vi "Main.vi"() -> ()   [LabVIEW 2024]
doc: "This template is for the Queued Message Handler design pattern.\n\nThe Event Handling Loop generates messages based on user interface actions.\n\nThe Message Handling Loop processes messages generated by the Event Handling Loop, or by other messages. The messages are string values, so new messages can be added easily to the Message Cases case structure in the Message Handling Loop. Each message cluster can also provide an optional value for Message Data, which is a variant that can be converted to whatever message-specific data is required."
uses:
  controls/UI Data.ctl
  support/Message Queue/Enqueue Message (Single).vi
  <vilib>/Utility/error.llb/Error Cluster From Error Code.vi
  <vilib>/ErrorRing/Error Ring.xnode
  support/Message Queue/Message Queue.lvlib
  support/User Event - Stop/User Event - Stop.lvlib
  01 Queues/User Events.lvlib
panel:
  out "Waveform Chart":dbl(graph)
  in  "Knob":dbl(knob) scale=0.0..10.0
  out "Letrero":string
  in  "Hacer otra Cosa":bool
  in  "Hacer Algo":bool
  in  "Sali":bool
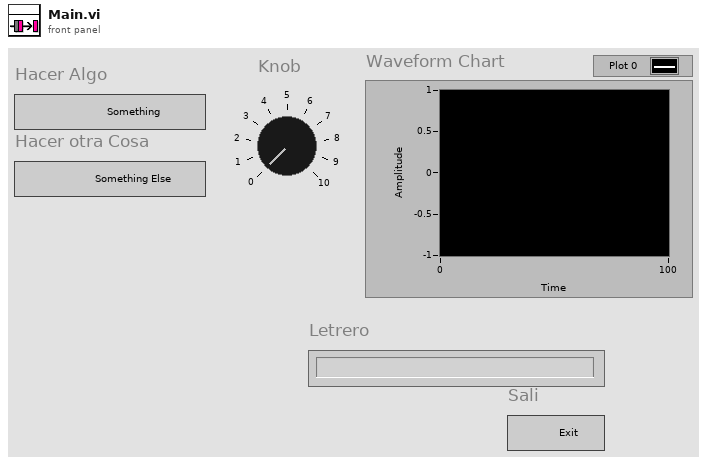
[diagram p1: front panel]
types:
  T1 = typedef "UI Data.ctl" = cluster{"Boolean <Replace Me>":bool, "String <Replace Me>":string, "Numeric <Replace Me>":dbl, "Do Something Ref":refnum<vi>, "Do Something Else Ref":refnum<vi>, "Data Display Ref":refnum<vi>, "Exit Button Ref":refnum<vi>}
  T2 = typedef "Message Queue.lvlib/All Message Queues.ctl" = cluster{"UI":refnum<queue>}
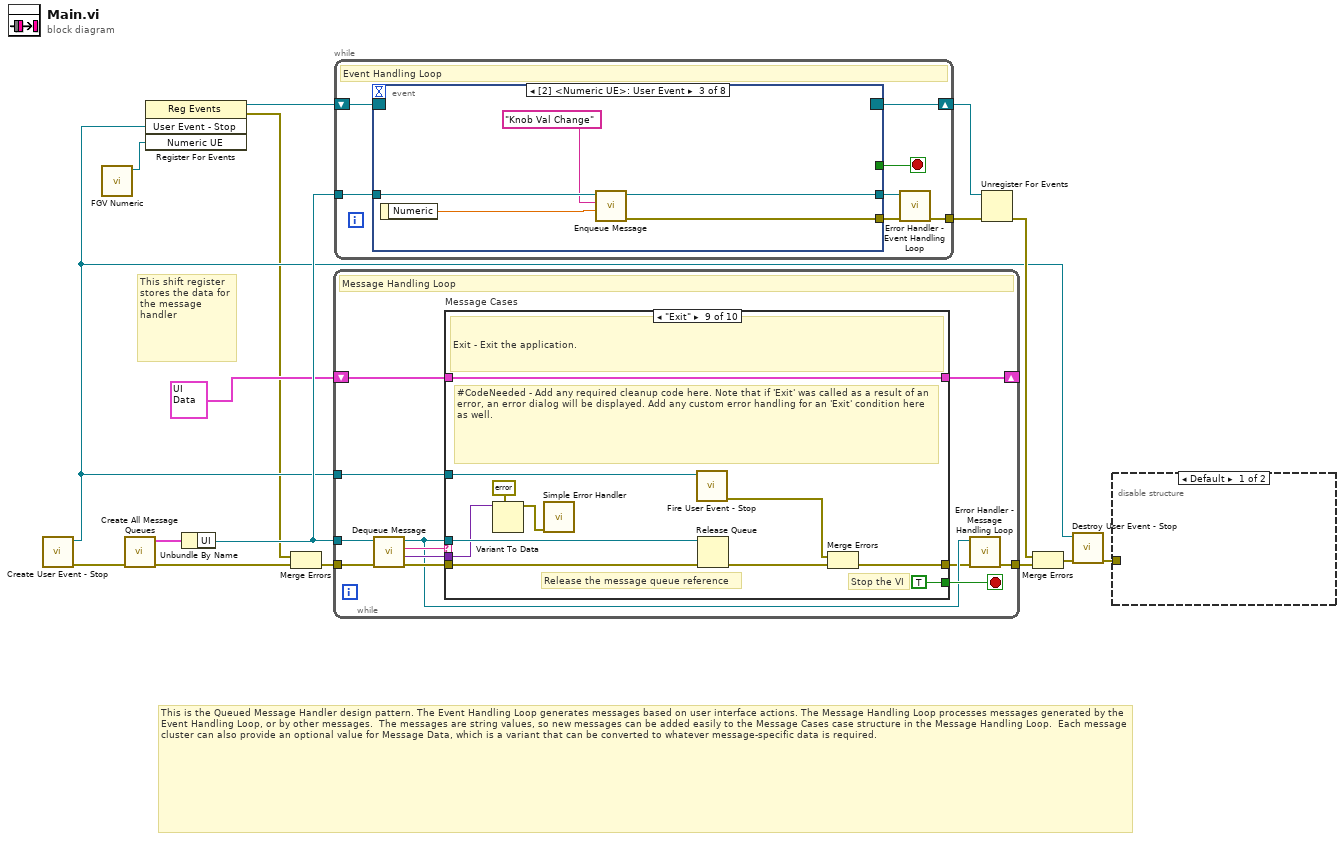
[diagram p0: block diagram]
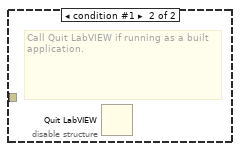
[diagram p2: hidden frame]
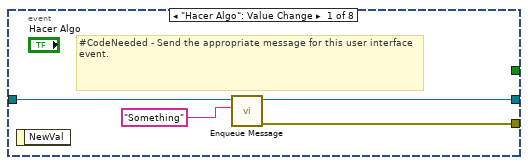
[diagram p3: hidden frame]
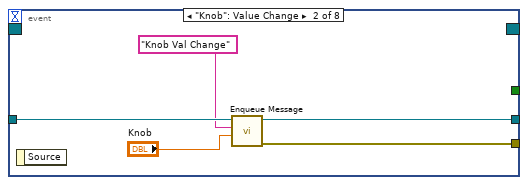
[diagram p4: hidden frame]
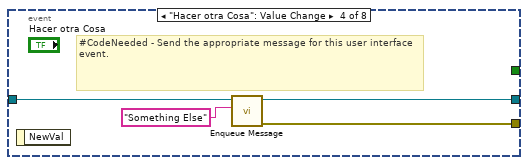
[diagram p5: hidden frame]
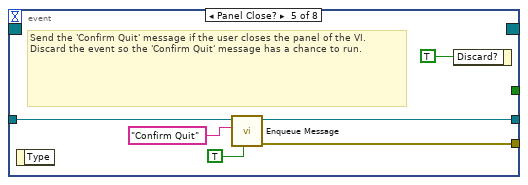
[diagram p6: hidden frame]
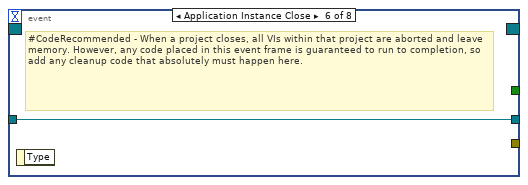
[diagram p7: hidden frame]
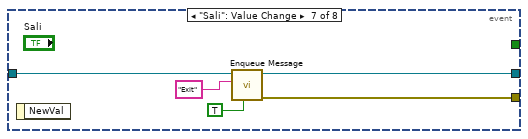
[diagram p8: hidden frame]
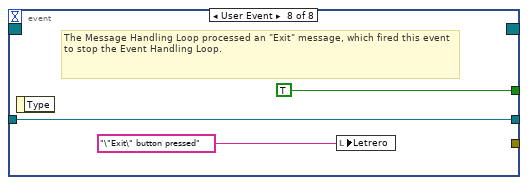
[diagram p9: hidden frame]
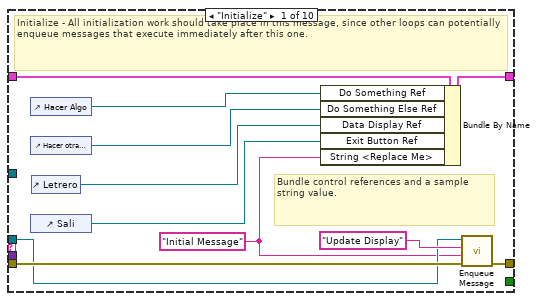
[diagram p10: hidden frame]
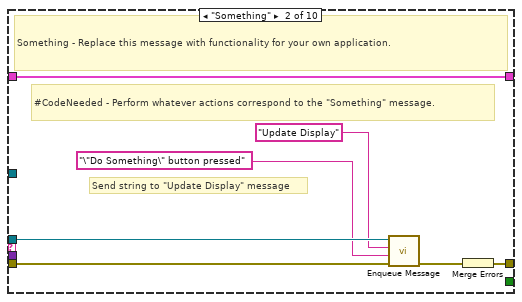
[diagram p11: hidden frame]
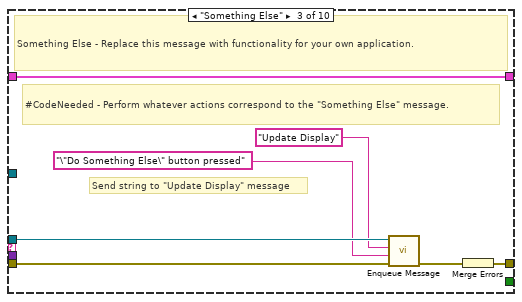
[diagram p12: hidden frame]
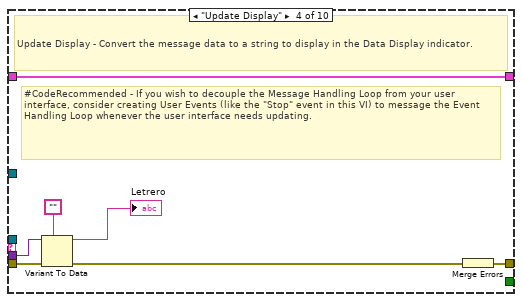
[diagram p13: hidden frame]
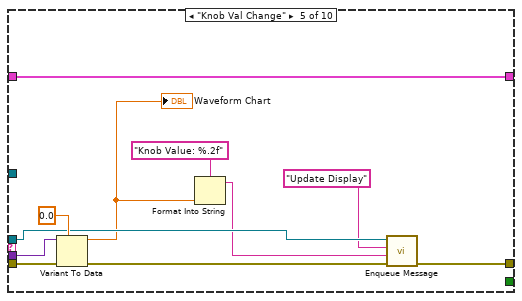
[diagram p14: hidden frame]
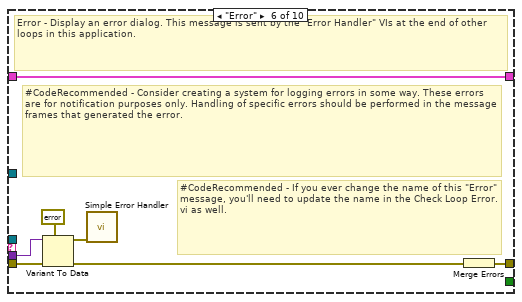
[diagram p15: hidden frame]
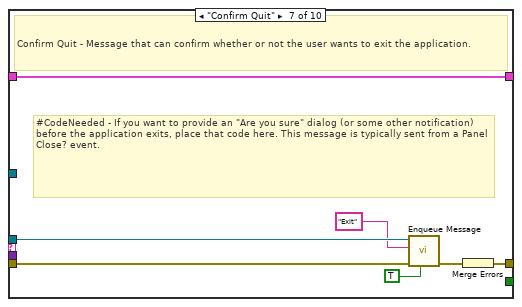
[diagram p16: hidden frame]
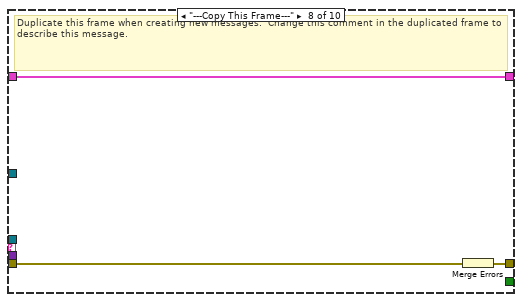
[diagram p17: hidden frame]
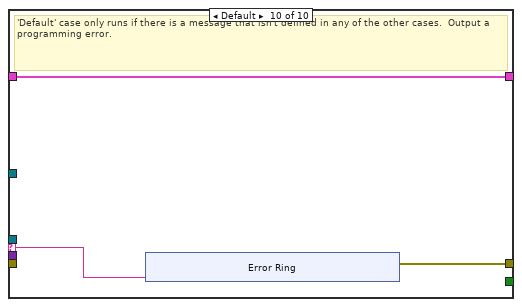
[diagram p18: hidden frame]
diagram:
  # "This is the Queued Message Handler design pattern. The Event Handling Loop generates messages based on user interface actions. The Message Handling Loop processes messages generated by the Event Handling Loop, or by other messages.  The messages are string values, so new messages can be added easily to the Message Cases case structure in the Message Handling Loop.  Each message cluster can also provide an optional value for Message Data, which is a variant that can be converted to whatever message-specific data is required."
  # "This shift register stores the data for the message handler"
  n1 = call "Create User Event - Stop.vi"() -> ("error out"=w12:errorcluster, "User Event - Stop"=w4:refnum<user-event>)  [unwired: 10 in]
  n2 = call "FGV Numeric.vi"() -> ("Numeric UE"=w1:refnum<user-event>)  [unwired: 11 in]
  n3 = call "Create All Message Queues.vi"("error in (no error)"=w12) -> ("error out"=w16:errorcluster, "Message Queues out"=w15:T2)  [unwired: 9 in]
  n4 = register-events(w4, w1) -> (reference out=w5:refnum<event-registration>, error out=w2:errorcluster)  [unwired: 2 in]
  n5 = Unbundle By Name(w15) -> ("UI"=w13:refnum<queue>)
  n6 = Merge Errors(w2, w16) -> (w3:errorcluster)
  n7 = while {
    tunnel: w13 -> [w20]
    shift-right: [w27] -> _
    shift-left: T1 {"Boolean <Replace Me>"=FALSE, "String <Replace Me>"="", "Numeric <Replace Me>"=0.0, "Do Something Ref"=refnum, "Do Something Else Ref"=refnum, "Data Display Ref"=refnum, "Exit Button Ref"=refnum} ("Data Cluster") -> [w28]
    tunnel: w4 -> [w25]
    tunnel: w3 -> [w24]
    tunnel: [w18] -> w14
    stop <- w26 stop-if-true
    # "Message Handling Loop"
    n8 = call "Dequeue Message.vi"("error in (no error)"=w24, "Message Queue"=w20) -> ("error out"=w23:errorcluster, "Message Data"=w21:variant, "Message"=w22:string, "dup Message Queue"=w19:refnum<queue>)  [unwired: 6 in]
    n9 = case "Message Cases" shown="\"Exit\"" w22 {
      selector: w22 -> [_ _ _ _ _ _ _ _ _ w100]
      tunnel: w19 -> [w30 w42 w49 _ w65 _ w81 _ w99 _]
      tunnel: w23 -> [w38 w44 w51 w58 w71 w78 w85 w88 w92 _]
      tunnel: [w39 w45 w52 w59 w66 w72 w83 w86 w95 w101] -> w17
      tunnel: w28 -> [w37 w46 w53 w60 w70 w77 w84 w87 w98 w102]
      tunnel: [w36 w46 w53 w60 w70 w77 w84 w87 w98 w102] -> w27
      tunnel: [_ _ _ _ _ _ _ _ TRUE _] -> w26
      tunnel: w21 -> [_ _ _ w57 w68 w76 _ _ w89 _]
      tunnel: w25 -> [_ _ _ _ _ _ _ _ w94 _]
      frame "Initialize" {
        w29 = "Initial Message" ("Initial Message")
        # "Bundle control references and a sample string value."
        # "Initialize - All initialization work should take place in this message, since other loops can potentially enqueue messages that execute immediately after this one."
        n10 = control-ref of="Hacer Algo"() -> (w35:refnum<vi>)
        n11 = control-ref of="Hacer otra Cosa"() -> (w34:refnum<vi>)
        n12 = control-ref of="Sali"() -> (w32:refnum<vi>)
        n13 = control-ref of="Letrero"() -> (w33:refnum<vi>)
        n14 = Bundle By Name(cluster=w37, "Do Something Ref"=w35, "Do Something Else Ref"=w34, "Data Display Ref"=w33, "Exit Button Ref"=w32, "String <Replace Me>"=w29) -> (w36:T1)
        n15 = call-poly "Enqueue Message.vi"("error in (no error)"=w38, "Message Data"=w29, "Message"="Update Display", "Message Queue"=w30) -> ("error out"=w39:errorcluster)  [unwired: 6 in, 1 out]
      }
      frame "Something" {
        # "Send string to \"Update Display\" message"
        # "#CodeNeeded - Perform whatever actions correspond to the \"Something\" message."
        # "Something - Replace this message with functionality for your own application."
        n16 = call-poly "Enqueue Message.vi"("error in (no error)"=w44, "Message Data"="\"Do Something\" button pressed" ("\"Do Something\" button pressed"), "Message"="Update Display", "Message Queue"=w42) -> ("error out"=w43:errorcluster)  [unwired: 6 in, 1 out]
        n17 = Merge Errors(w43) -> (w45:errorcluster)
      }
      frame "Something Else" {
        # "Send string to \"Update Display\" message"
        # "#CodeNeeded - Perform whatever actions correspond to the \"Something Else\" message."
        # "Something Else - Replace this message with functionality for your own application."
        n18 = call-poly "Enqueue Message.vi"("error in (no error)"=w51, "Message Data"="\"Do Something Else\" button pressed" ("\"Do Something Else\" button pressed"), "Message"="Update Display", "Message Queue"=w49) -> ("error out"=w50:errorcluster)  [unwired: 6 in, 1 out]
        n19 = Merge Errors(w50) -> (w52:errorcluster)
      }
      frame "Update Display" {
        # "#CodeRecommended - If you wish to decouple the Message Handling Loop from your user interface, consider creating User Events (like the \"Stop\" event in this VI) to message the Event Handling Loop whenever the user interface needs updating."
        # "Update Display - Convert the message data to a string to display in the Data Display indicator."
        n20 = Variant To Data(error in=w58, type="", Variant=w57) -> (data=→"Letrero":string, error out=w55:errorcluster)
        n21 = Merge Errors(w55) -> (w59:errorcluster)
      }
      frame "Knob Val Change" {
        n22 = Variant To Data(error in=w71, type=0.0, Variant=w68) -> (data=w62:dbl, error out=w69:errorcluster)
        "Waveform Chart" <- w62
        n23 = Format Into String(format string="Knob Value: %.2f", w62) -> (resulting string=w63:string)  [unwired: 2 in, 1 out]
        n24 = call-poly "Enqueue Message.vi"("error in (no error)"=w69, "Message Data"=w63, "Message"="Update Display", "Message Queue"=w65) -> ("error out"=w66:errorcluster)  [unwired: 6 in, 1 out]
      }
      frame "Error" {
        # "#CodeRecommended - If you ever change the name of this \"Error\" message, you'll need to update the name in the Check Loop Error.vi as well."
        # "#CodeRecommended - Consider creating a system for logging errors in some way. These errors are for notification purposes only. Handling of specific errors should be performed in the message frames that generated the error."
        # "Error - Display an error dialog. This message is sent by the \"Error Handler\" VIs at the end of other loops in this application."
        n25 = Variant To Data(error in=w78, type=errorcluster {"status"=FALSE, "code"=0, "source"=""} ("error constant"), Variant=w76) -> (data=w74:errorcluster, error out=w73:errorcluster)
        n26 = call <vilib>:"Simple Error Handler.vi"("error in (no error)"=w74) -> ()  [unwired: 4 in, 5 out]
        n27 = Merge Errors(w73) -> (w72:errorcluster)
      }
      frame "Confirm Quit" {
        # "#CodeNeeded - If you want to provide an \"Are you sure\" dialog (or some other notification) before the application exits, place that code here. This message is typically sent from a Panel Close? event."
        # "Confirm Quit - Message that can confirm whether or not the user wants to exit the application."
        n28 = call-poly "Enqueue Message.vi"("Priority Message? (F)"=TRUE, "error in (no error)"=w85, "Message"="Exit", "Message Queue"=w81) -> ("error out"=w82:errorcluster)  [unwired: 6 in, 1 out]
        n29 = Merge Errors(w82) -> (w83:errorcluster)
      }
      frame "---Copy This Frame---" {
        # "Duplicate this frame when creating new messages.  Change this comment in the duplicated frame to describe this message."
        n30 = Merge Errors(w88) -> (w86:errorcluster)
      }
      frame "Exit" {
        # "Stop the VI"
        # "Release the message queue reference"
        # "#CodeNeeded - Add any required cleanup code here. Note that if 'Exit' was called as a result of an error, an error dialog will be displayed. Add any custom error handling for an 'Exit' condition here as well."
        # "Exit - Exit the application."
        n31 = Variant To Data(type=errorcluster {"status"=FALSE, "code"=0, "source"=""} ("error constant"), Variant=w89) -> (data=w90:errorcluster)  [unwired: 1 in, 1 out]
        n32 = call <vilib>:"Simple Error Handler.vi"("error in (no error)"=w90) -> ()  [unwired: 4 in, 5 out]
        n33 = call "Fire User Event - Stop.vi"("User Event - Stop"=w94) -> ("error out"=w93:errorcluster)  [unwired: 10 in]
        n34 = Release Queue(queue=w99, error in (no error)=w92) -> (error out=w96:errorcluster)  [unwired: 1 in, 2 out]
        n35 = Merge Errors(w93, w96) -> (w95:errorcluster)
      }
      frame Default {
        # "'Default' case only runs if there is a message that isn't defined in any of the other cases.  Output a programming error."
        n36 = xnode "Error Ring"("parameter 0"=w100) -> ("error out"=w101:errorcluster)
      }
    }
    n37 = call "Error Handler - Message Handling Loop.vi"("error in (no error)"=w17, "Message Queue"=w19) -> ("dup error in"=w18:errorcluster)  [unwired: 8 in, 1 out]
  }
  n38 = while {
    tunnel: w13 -> [w116]
    shift-right: [w114] -> w9
    shift-left: w5 -> [w115]
    tunnel: [w110] -> w6
    stop <- w112 stop-if-true
    # "Event Handling Loop"
    n39 = event shown="[2] <Numeric UE>: User Event" {
      selector: w115 -> [_ _ _ _ _ _ _ _]
      dyn-events: [_ _ _ _ _ _ _ _] -> w114
      timeout: _ -> [_ _ _ _ _ _ _ _]
      tunnel: [_ _ _ _ _ _ _ TRUE ("Discard?")] -> w112
      tunnel: w116 -> [w120 w125 w130 w134 w139 w141 w146 w149]
      tunnel: [w117 w122 w127 w131 w138 _ w145 _] -> w113
      tunnel: [w119 w124 w129 w133 w137 w141 w144 w149] -> w111
      event "Hacer Algo": Value Change {
        # "#CodeNeeded - Send the appropriate message for this user interface event."
        n40 = event-data() -> ()  [unwired: 1 in, 1 out]
        n41 = call-poly "Enqueue Message.vi"("Message"="Something", "Message Queue"=w120) -> ("error out"=w117:errorcluster, "dup Message Queue"=w119:refnum<queue>)  [unwired: 8 in]
      }
      event "Knob": Value Change {
        n42 = event-data() -> ()  [unwired: 1 in, 1 out]
        n43 = call-poly "Enqueue Message.vi"("Message Data"="Knob", "Message"="Knob Val Change", "Message Queue"=w125) -> ("error out"=w122:errorcluster, "dup Message Queue"=w124:refnum<queue>)  [unwired: 7 in]
      }
      event User Event {
        n44 = event-data() -> ("Numeric"=w126:dbl)  [unwired: 1 in]
        n45 = call-poly "Enqueue Message.vi"("Message Data"=w126, "Message"="Knob Val Change", "Message Queue"=w130) -> ("error out"=w127:errorcluster, "dup Message Queue"=w129:refnum<queue>)  [unwired: 7 in]
      }
      event "Hacer otra Cosa": Value Change {
        # "#CodeNeeded - Send the appropriate message for this user interface event."
        n46 = event-data() -> ()  [unwired: 1 in, 1 out]
        n47 = call-poly "Enqueue Message.vi"("Message"="Something Else", "Message Queue"=w134) -> ("error out"=w131:errorcluster, "dup Message Queue"=w133:refnum<queue>)  [unwired: 8 in]
      }
      event Panel Close? {
        # "Send the 'Confirm Quit' message if the user closes the panel of the VI. Discard the event so the 'Confirm Quit' message has a chance to run."
        n48 = event-data() -> ()  [unwired: 1 in, 1 out]
        n49 = call-poly "Enqueue Message.vi"("Priority Message? (F)"=TRUE, "Message"="Confirm Quit", "Message Queue"=w139) -> ("error out"=w138:errorcluster, "dup Message Queue"=w137:refnum<queue>)  [unwired: 7 in]
        n50 = event-data("Discard?"=TRUE) -> ()  [unwired: 1 in, 1 out]
      }
      event Application Instance Close {
        # "#CodeRecommended - When a project closes, all VIs within that project are aborted and leave memory. However, any code placed in this event frame is guaranteed to run to completion, so add any cleanup code that absolutely must happen here."
        n51 = event-data() -> ()  [unwired: 1 in, 1 out]
      }
      event "Sali": Value Change {
        n52 = event-data() -> ()  [unwired: 1 in, 1 out]
        n53 = call-poly "Enqueue Message.vi"("Priority Message? (F)"=TRUE, "Message"="Exit", "Message Queue"=w146) -> ("error out"=w145:errorcluster, "dup Message Queue"=w144:refnum<queue>)  [unwired: 7 in]
      }
      event User Event {
        # "The Message Handling Loop processed an \"Exit\" message, which fired this event to stop the Event Handling Loop."
        n54 = event-data() -> ()  [unwired: 1 in, 1 out]
        n55 = local write "Letrero"("\"Exit\" button pressed" ("VI Stopped")) -> ()
      }
    }
    n56 = call "Error Handler - Event Handling Loop.vi"("error in (no error)"=w113, "Message Queue"=w111) -> ("dup error in"=w110:errorcluster)  [unwired: 8 in, 1 out]
  }
  n57 = Unregister For Events(event registration refnum=w9, error in=w6) -> (error out=w10:errorcluster)
  n58 = Merge Errors(w10, w14) -> (w11:errorcluster)
  n59 = call "Destroy User Event - Stop.vi"("error in (no error)"=w11, "User Event - Stop"=w4) -> ("error out"=w7:errorcluster)  [unwired: 9 in]
  n60 = disable-structure shown="Default" {
    disable-tunnel: w7 -> [_ _]
    frame condition #0 (active) {
    }
    frame condition #1 {
      # "Call Quit LabVIEW if running as a built application."
      n61 = Quit LabVIEW() -> ()  [unwired: 1 in]
    }
  }
